vi "Calculate True Y Position.vi"(8 "error in (no error)":errorcluster, 10 "Y Position":dbl format="%#_13g", 11 "Program Data":T2 {"Time"."Time/Div" min=0.0 max=16.0 step=1.0 scale=0.0..12.0; "CH1"."Vertical Position (Div)" min=-5.0 max=5.0 step=0.1 scale=-5.0..5.0; "CH1"."Volts/Div" min=0 max=8 step=1 scale=0.0..8.0; "CH0"."Vertical Position (Div)" min=-5.0 max=5.0 step=0.1 scale=-5.0..5.0; "CH0"."Volts/Div" min=0 max=8 step=1 scale=0.0..8.0; "Wave Parameters"."Phase offset (deg)" format="%#_6p"; "Wave Parameters"."Frequency (Hz)" format="%#_6p"}) -> (0 "error out":errorcluster, 1 "Units":string, 2 "True Y Position":T1 min=-5.0 max=5.0 step=0.1 scale=-5.0..5.0, 3 "Program Data Out":T2 {"Time"."Time/Div" min=0.0 max=16.0 step=1.0 scale=0.0..12.0; "CH1"."Vertical Position (Div)" min=-5.0 max=5.0 step=0.1 scale=-5.0..5.0; "CH1"."Volts/Div" min=0 max=8 step=1 scale=0.0..8.0; "CH0"."Vertical Position (Div)" min=-5.0 max=5.0 step=0.1 scale=-5.0..5.0; "CH0"."Volts/Div" min=0 max=8 step=1 scale=0.0..8.0; "Wave Parameters"."Phase offset (deg)" format="%#_6p"; "Wave Parameters"."Frequency (Hz)" format="%#_6p"})   [LabVIEW 2021]
uses:
  Controls/Program Data.ctl
  Controls/Measurements.ctl
  Controls/Channel Measurement String Control.ctl
  Controls/Cursor Info.ctl
  Controls/Communication Cluster.ctl
  <vilib>/NI/STM/TCP/TCP Connection Info.ctl
  <vilib>/NI/STM/SubVIs/MetaDataElement.ctl
  Communication/Scope Data.ctl
  Program Files (x86)/National Instruments/LabVIEW 2021/ProjectTemplates/Source/myRIO/Oscilloscope/myRIO v1.1/Real-Time/Controls/Wave Parameters.ctl
  Program Files (x86)/National Instruments/LabVIEW 2021/ProjectTemplates/Source/myRIO/Oscilloscope/myRIO v1.1/Real-Time/Controls/Waveform Enum.ctl
  Program Files (x86)/National Instruments/LabVIEW 2021/ProjectTemplates/Source/myRIO/Oscilloscope/myRIO v1.1/Real-Time/Controls/Channel Selector.ctl
  Controls/Channel Settings.ctl
  Controls/Analog Input Selector.ctl
  Controls/Knob.ctl
  Controls/Vertical Position.ctl
  Controls/Channel Parameters.ctl
  Controls/Time Selector.ctl
  Controls/Time Knob.ctl
  Controls/FGen Desktop Configuration.ctl
  <vilib>/NI/STM/NI STM.lvlib
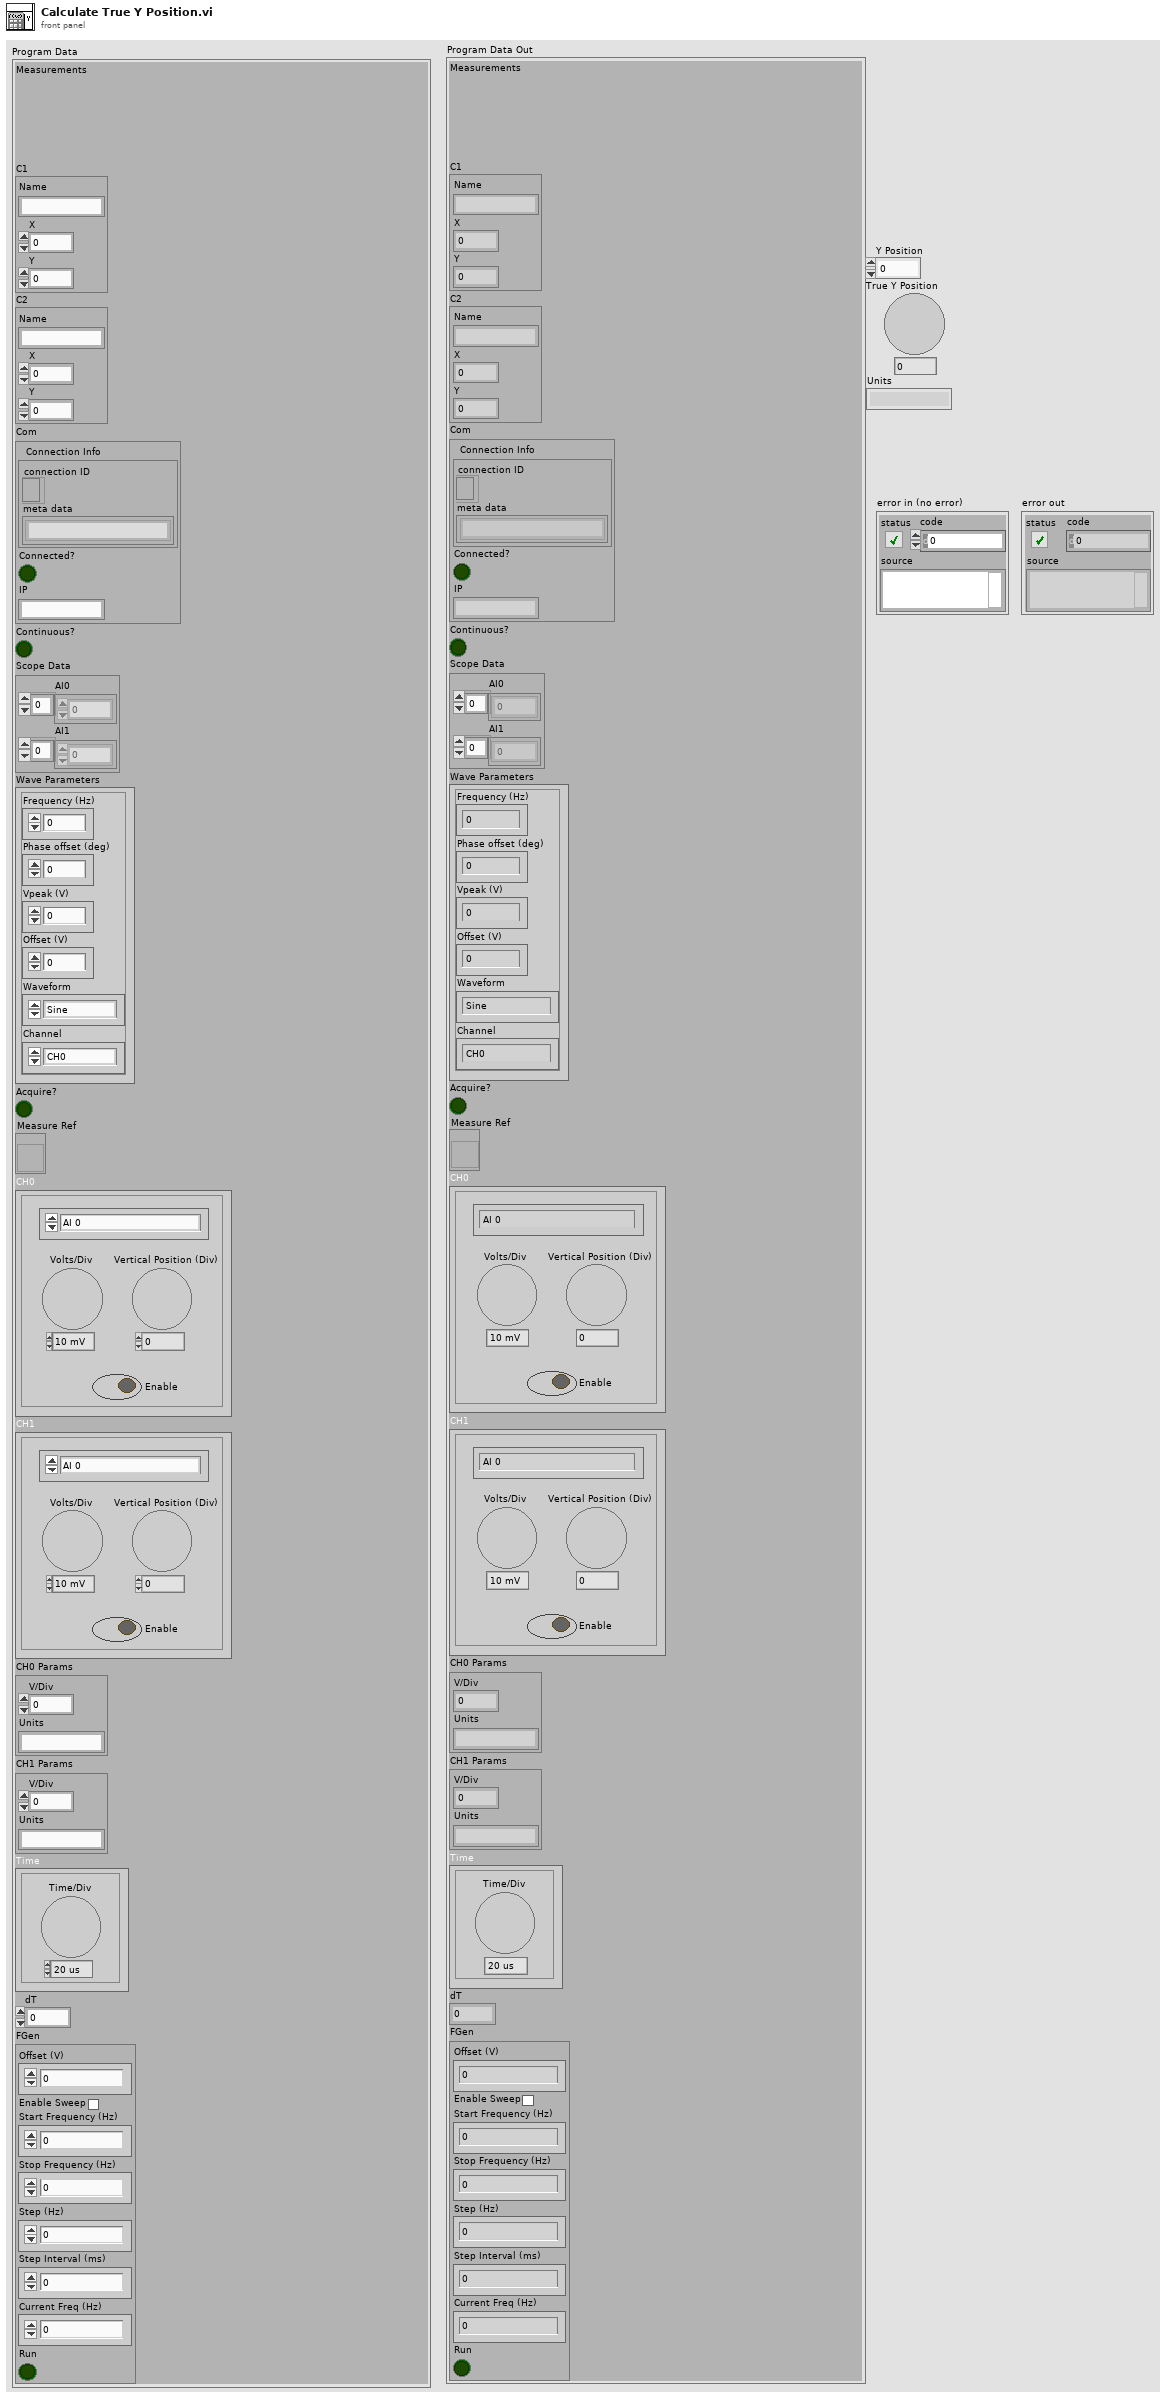
[diagram p1: front panel]
types:
  T1 = typedef "Vertical Position.ctl" = dbl
  T2 = typedef "Program Data.ctl" = cluster{"Measurements":T3, "C1":T5, "C2":T5, "Com":T6, "Continuous?":bool, "Scope Data":T9, "Wave Parameters":T10, "Acquire?":bool, "Measure Ref":refnum<vi>, "CH0":T13, "CH1":T13, "CH0 Params":T16, "CH1 Params":T16, "Time":T17, "dT":dbl, "FGen":T19}
  T3 = typedef "Measurements.ctl" = cluster{"Channel 0":T4, "RMS 0":T4, "Vp-p 0":T4, "Freq 0":T4, "Channel 1":T4, "RMS 1":T4, "Vp-p 1":T4, "Freq 1":T4, "Cursors":T4, "C1":T4, "C2":T4, "dT":T4}
  T4 = typedef "Channel Measurement String Control.ctl" = string
  T5 = typedef "Cursor Info.ctl" = cluster{"Name":string, "X":dbl, "Y":dbl}
  T6 = typedef "Communication Cluster.ctl" = cluster{"Connection Info":T7, "Connected?":bool, "IP":string}
  T7 = typedef "NI STM.lvlib/TCP Connection Info.ctl" = cluster{"connection ID":refnum<k5>, "meta data":T8[]}
  T8 = typedef "NI STM.lvlib/MetaDataElement.ctl" = string
  T9 = typedef "Scope Data.ctl" = cluster{"AI0":dbl[], "AI1":dbl[]}
  T10 = typedef "Wave Parameters.ctl" = cluster{"Frequency (Hz)":dbl, "Phase offset (deg)":dbl, "Vpeak (V)":dbl, "Offset (V)":dbl, "Waveform":T11, "Channel":T12}
  T11 = typedef "Waveform Enum.ctl" = enum16{"Sine", "Square"}
  T12 = typedef "Channel Selector.ctl" = enum16{"CH0", "CH1"}
  T13 = typedef "Channel Settings.ctl" = cluster{"Channel":T14, "Enable":bool, "Volts/Div":T15, "Vertical Position (Div)":T1}
  T14 = typedef "Analog Input Selector.ctl" = enum16{"AI 0", "AI 1"}
  T15 = typedef "Knob.ctl" = i32
  T16 = typedef "Channel Parameters.ctl" = cluster{"V/Div":dbl, "Units":string}
  T17 = typedef "Time Selector.ctl" = cluster{"Time/Div":T18}
  T18 = typedef "Time Knob.ctl" = dbl
  T19 = typedef "FGen Desktop Configuration.ctl" = cluster{"Offset (V)":dbl, "Enable Sweep":bool, "Start Frequency (Hz)":dbl, "Stop Frequency (Hz)":dbl, "Step (Hz)":dbl, "Step Interval (ms)":dbl, "Current Freq (Hz)":dbl, "Run":bool}
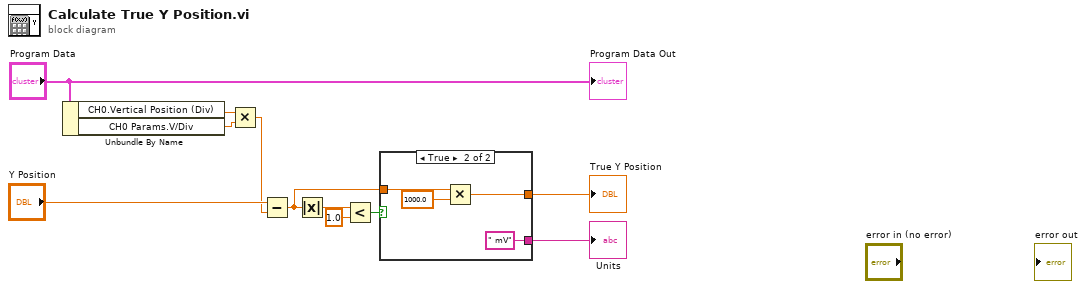
[diagram p0: block diagram]
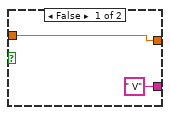
[diagram p2: hidden frame]
diagram:
  n1 = Unbundle By Name("Program Data") -> ("CH0.Vertical Position (Div)"=w10:T1, "CH0 Params.V/Div"=w11:dbl)
  n2 = Multiply(x=w10, y=w11) -> (x*y=w7:T1)
  n3 = Subtract(x="Y Position", y=w7) -> (x-y=w4:T1)
  n4 = Absolute Value(x=w4) -> (abs(x)=w1:T1)
  n5 = Less?(x=w1, y=T1 1.0) -> (x < y?=w5:bool)
  n6 = case shown="True" w5 {
    tunnel: w4 -> [w13 w17]
    tunnel: [w13 w15] -> w3
    tunnel: [" V" " mV"] -> w2
    frame False {
    }
    frame True {
      n7 = Multiply(x=w17, y=T1 1000.0) -> (x*y=w15:T1)
    }
  }
  "True Y Position" <- w3
  "Units" <- w2
  "Program Data Out" <- "Program Data"
